vi "Initialize_Devices.vi"(6 "Queues":T3, 8 "Status/Errors in":refnum<vi>, 9 "Control Parameters [] in":T18[](array[typedef]) {"Aux Byte Value" format="%02x"; "Max Real Value" format="%#_6e"; "Min Real Value" format="%#_6e"; "dReal/dByte" format="%#_6e"; "Byte Value" format="%02x"; "Identifier" format="%02x"}, 10 "Main parameters in":T4={"Mode"={"Mode"=enum."Dialog", "Expert?"=FALSE, "Dialog?"=FALSE}, "Stop loop"={"Settings changed?"=FALSE, "Stop?"=refnum}, "Send message"={"Send mode"=enum."Get parameters", "Set parameter list"=0, "Get parameter list"=0, "Reset device"=0, "Length set settings message"=0, "Reset buttons?"=FALSE, "Reset Master?"=enum."General"}, "Write settings"={"Options"=enum."File 1"}, "Settings state"={"MAS locked?"=refnum, "SLV locked?"=refnum}, "Button refs"={"Stop program"=refnum, "Save settings"=refnum, "DAQ mode"=refnum, "Reset settings"=refnum, "Apply settings"=refnum, "Reset MAS"=refnum, "Reset SLV"=refnum, "Local DBase?"=refnum, "Last value DBase"=FALSE, "Database"=refnum, "Calibration"=refnum, "Save settings 2"=refnum}, "Update screen"={"Detector number"=0, "Hardware"=enum."None"}, "Files"={"Path config file"=path "", "Path def. ini file"=path "", "Path ini file 1"=path "", "Path ini file 2"=path "", "Path RBF file"=path ""}, "DB connection"={"connection reference"=refnum, "Connected?"=refnum, "ODBC Name"=""}, "Status_id"=refnum, "Time difference"=refnum, "Satellites"=refnum, "Alignment parameters"=refnum, "Page Statistics 2"=refnum, "Database"=refnum, "Page Statistics"=refnum} {"Update screen"."Detector number" format="%#.0f"; "Send message"."Reset device" format="%x"; "Send message"."Get parameter list" format="%x"; "Send message"."Set parameter list" format="%x"}, 11 "Timer parameters":refnum<vi>) -> (0 "Status/Errors out":refnum<vi>, 1 "Control Parameters [] out":T18[](array[typedef]) {"Aux Byte Value" format="%02x"; "Max Real Value" format="%#_6e"; "Min Real Value" format="%#_6e"; "dReal/dByte" format="%#_6e"; "Byte Value" format="%02x"; "Identifier" format="%02x"}, 2 "Main parameters out":T4={"Mode"={"Mode"=enum."Dialog", "Expert?"=FALSE, "Dialog?"=FALSE}, "Stop loop"={"Settings changed?"=FALSE, "Stop?"=refnum}, "Send message"={"Send mode"=enum."Get parameters", "Set parameter list"=0, "Get parameter list"=0, "Reset device"=0, "Length set settings message"=0, "Reset buttons?"=FALSE, "Reset Master?"=enum."General"}, "Write settings"={"Options"=enum."File 1"}, "Settings state"={"MAS locked?"=refnum, "SLV locked?"=refnum}, "Button refs"={"Stop program"=refnum, "Save settings"=refnum, "DAQ mode"=refnum, "Reset settings"=refnum, "Apply settings"=refnum, "Reset MAS"=refnum, "Reset SLV"=refnum, "Local DBase?"=refnum, "Last value DBase"=FALSE, "Database"=refnum, "Calibration"=refnum, "Save settings 2"=refnum}, "Update screen"={"Detector number"=0, "Hardware"=enum."None"}, "Files"={"Path config file"=path "", "Path def. ini file"=path "", "Path ini file 1"=path "", "Path ini file 2"=path "", "Path RBF file"=path ""}, "DB connection"={"connection reference"=refnum, "Connected?"=refnum, "ODBC Name"=""}, "Status_id"=refnum, "Time difference"=refnum, "Satellites"=refnum, "Alignment parameters"=refnum, "Page Statistics 2"=refnum, "Database"=refnum, "Page Statistics"=refnum} {"Update screen"."Detector number" format="%#.0f"; "Send message"."Reset device" format="%x"; "Send message"."Get parameter list" format="%x"; "Send message"."Set parameter list" format="%x"}, 3 "Devices":T17)   [LabVIEW 2010]
uses:
  Controls/Control_Parameters.ctl
  Controls/Master.ctl
  Controls/Devices.ctl
  Controls/Main_Parameters.ctl
  Controls/Mode.ctl
  Controls/Stop_Loop.ctl
  Controls/Send_Message.ctl
  Controls/Send_Message_Mode.ctl
  Controls/Write_Settings.ctl
  Controls/Write_Settings_Options.ctl
  Controls/Settings_State.ctl
  Controls/Button_Refs.ctl
  Controls/Update_Screen.ctl
  Controls/Files.ctl
  Controls/DB_Connection.ctl
  database/Connection.llb/Conn ObjectReference.ctl
  Controls/Queues.ctl
  Controls/One_Second.ctl
  Controls/GPS_Timestamp.ctl
  Controls/Device.ctl
  Controls/Set_Mode.ctl
  Controls/Get_Set_Connection_Options.ctl
  Controls/Get_Set_Buttons_mode.ctl
  Controls/Get_Set_Settings_State_Options.ctl
panel:
  in  "Slave":T1
  in  "Master":T1
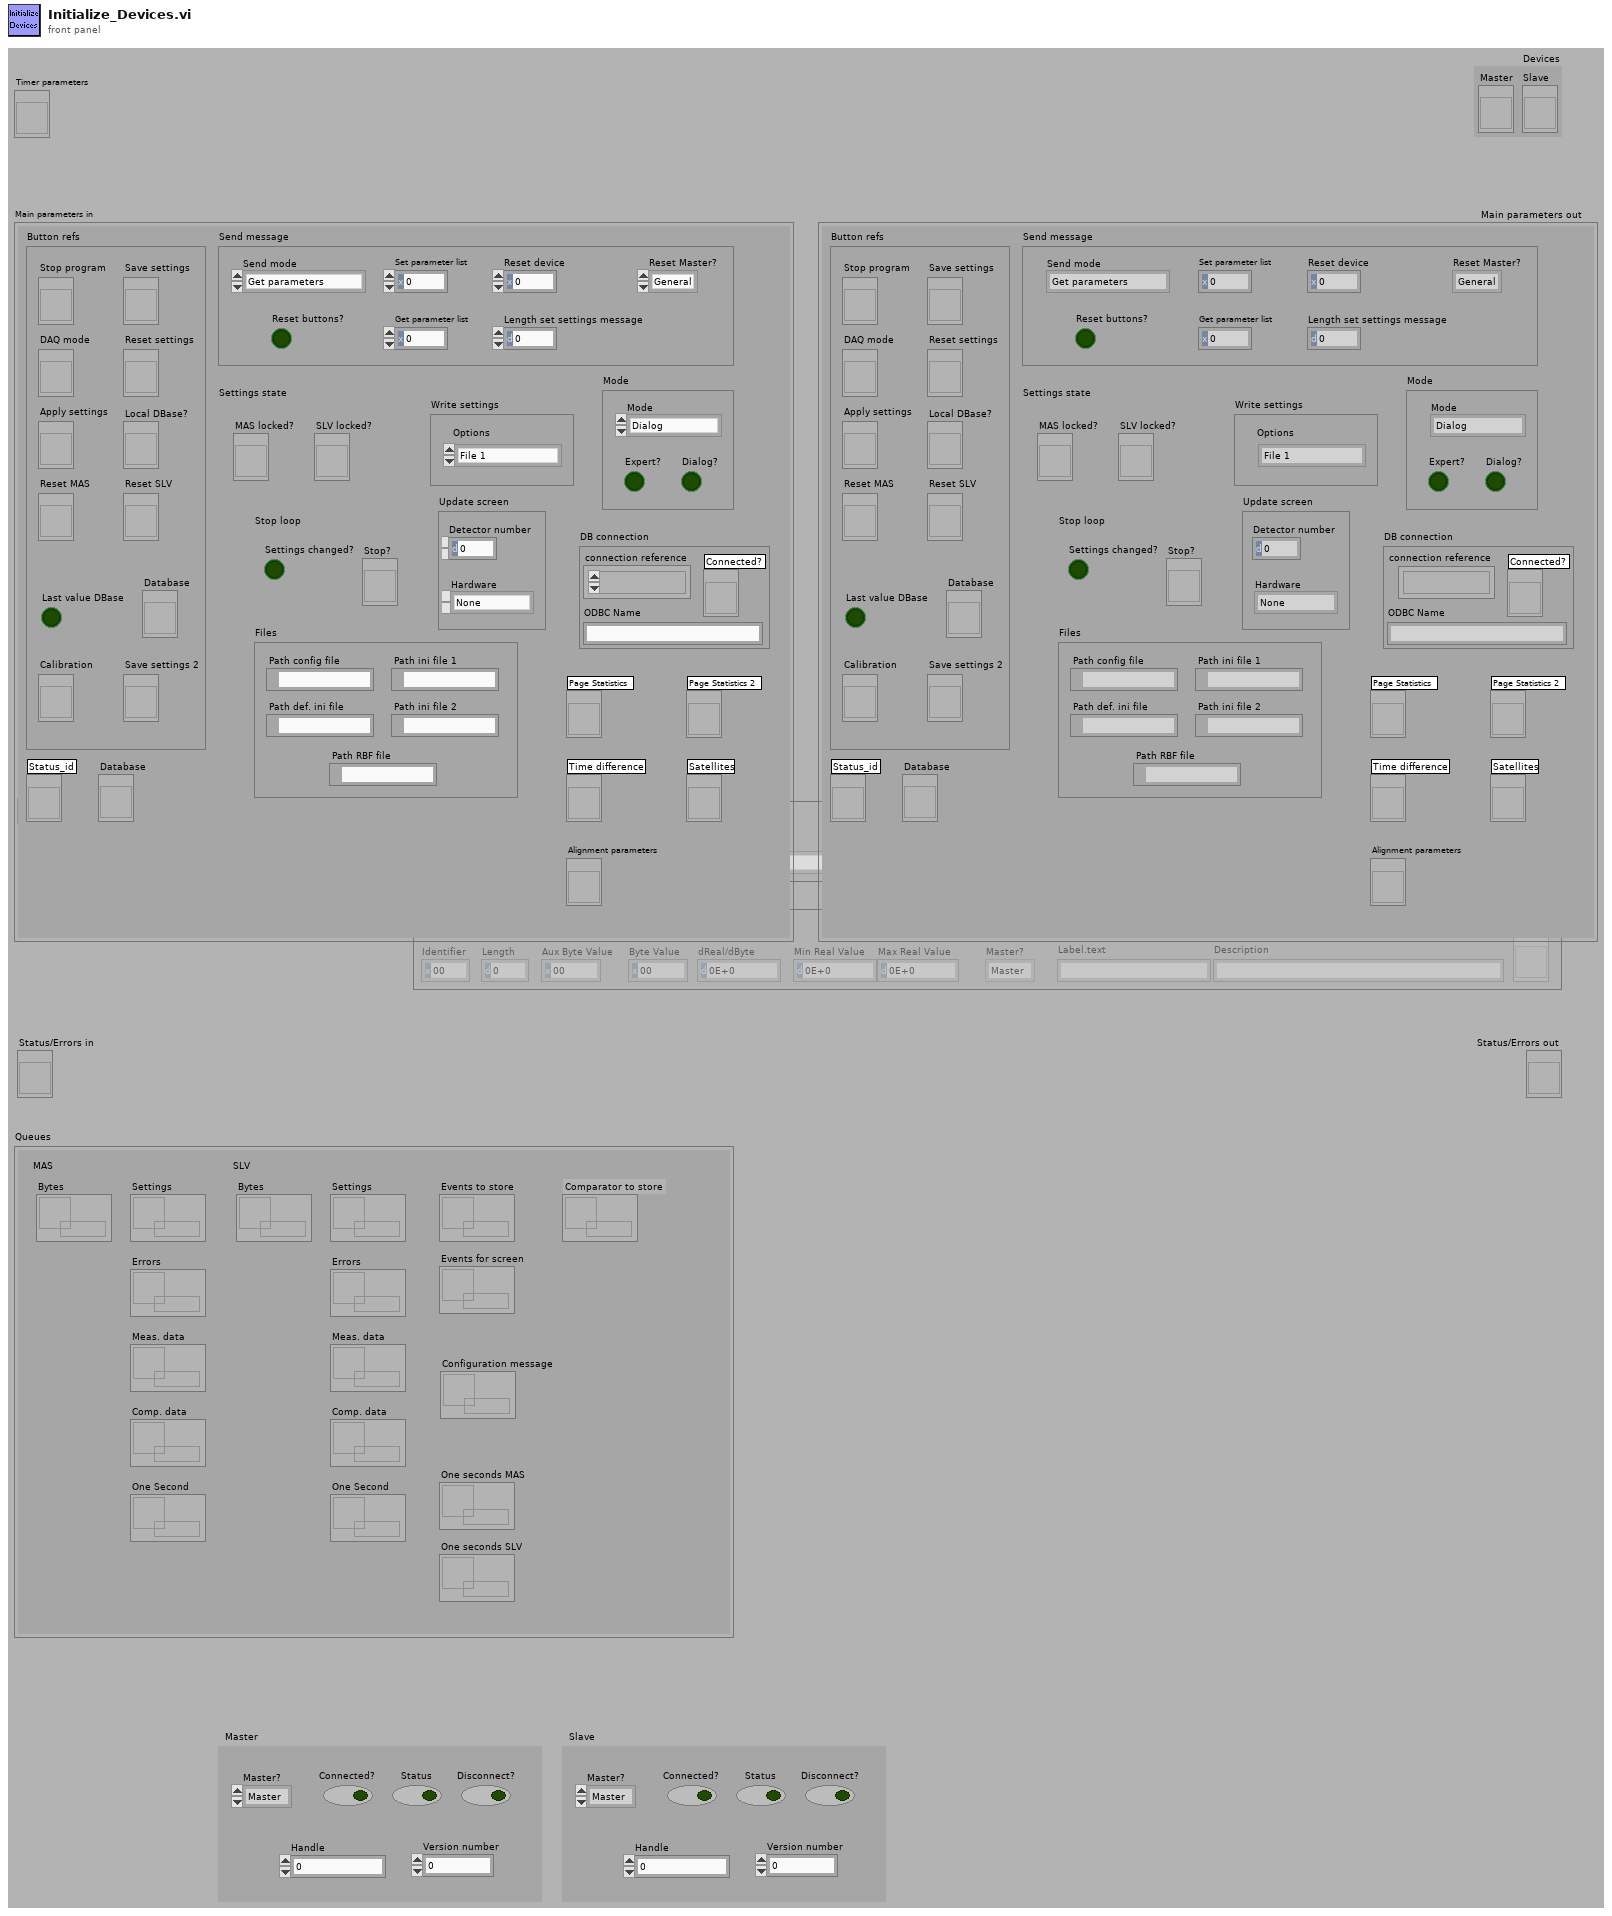
[diagram p1: front panel]
types:
  T1 = typedef "Device.ctl" = cluster{"Master?":T2, "Connected?":bool, "Status":bool, "Disconnect?":bool, "Handle":u32, "Version number":u32}
  T2 = typedef "Master.ctl" = enum16{"Master", "Slave", "General"}
  T3 = typedef "Queues.ctl" = cluster{"MAS":cluster{"Bytes":refnum<queue>, "Settings":refnum<queue>, "Errors":refnum<queue>, "Meas. data":refnum<queue>, "One Second":refnum<queue>, "Comp. data":refnum<queue>}, "SLV":cluster{"Bytes":refnum<queue>, "Settings":refnum<queue>, "Errors":refnum<queue>, "Meas. data":refnum<queue>, "One Second":refnum<queue>, "Comp. data":refnum<queue>}, "Events to store":refnum<queue>, "Events for screen":refnum<queue>, "One seconds MAS":refnum<queue>, "One seconds SLV":refnum<queue>, "Configuration message":refnum<queue>, "Comparator to store":refnum<queue>}
  T4 = typedef "Main_Parameters.ctl" = cluster{"Mode":T5, "Stop loop":T6, "Send message":T7, "Write settings":T9, "Settings state":T11, "Button refs":T12, "Update screen":T13, "Files":T14, "DB connection":T15, "Status_id":refnum<vi>, "Time difference":refnum<vi>, "Satellites":refnum<vi>, "Alignment parameters":refnum<vi>, "Page Statistics 2":refnum<vi>, "Database":refnum<vi>, "Page Statistics":refnum<vi>}
  T5 = typedef "Mode.ctl" = cluster{"Mode":enum8{"Stop", "Dialog", "Hisparc II", "Hisparc II DAQ", "Alignment"}, "Expert?":bool, "Dialog?":bool}
  T6 = typedef "Stop_Loop.ctl" = cluster{"Settings changed?":bool, "Stop?":refnum<vi>}
  T7 = typedef "Send_Message.ctl" = cluster{"Send mode":T8, "Set parameter list":u8, "Get parameter list":u8, "Reset device":u8, "Length set settings message":i32, "Reset buttons?":bool, "Reset Master?":T2}
  T8 = typedef "Send_Message_Mode.ctl" = enum16{"Get parameters", "Set parameters", "From front panel", "From parameters", "Reset device", "Alignment"}
  T9 = typedef "Write_Settings.ctl" = cluster{"Options":T10}
  T10 = typedef "Write_Settings_Options.ctl" = enum16{"File 1", "File 2", "Alignment", "Reset"}
  T11 = typedef "Settings_State.ctl" = cluster{"MAS locked?":refnum<vi>, "SLV locked?":refnum<vi>}
  T12 = typedef "Button_Refs.ctl" = cluster{"Stop program":refnum<vi>, "Save settings":refnum<vi>, "DAQ mode":refnum<vi>, "Reset settings":refnum<vi>, "Apply settings":refnum<vi>, "Reset MAS":refnum<vi>, "Reset SLV":refnum<vi>, "Local DBase?":refnum<vi>, "Last value DBase":bool, "Database":refnum<vi>, "Calibration":refnum<vi>, "Save settings 2":refnum<vi>}
  T13 = typedef "Update_Screen.ctl" = cluster{"Detector number":u16, "Hardware":enum8{"None", "HiSPARC I", "HiSPARC II", "HiSPARC III", "Unknown"}}
  T14 = typedef "Files.ctl" = cluster{"Path config file":path, "Path def. ini file":path, "Path ini file 1":path, "Path ini file 2":path, "Path RBF file":path}
  T15 = typedef "DB_Connection.ctl" = cluster{"connection reference":T16, "Connected?":refnum<vi>, "ODBC Name":string}
  T16 = typedef "Conn ObjectReference.ctl" = refnum<k1>
  T17 = typedef "Devices.ctl" = cluster{"Master":refnum<vi>, "Slave":refnum<vi>}
  T18 = typedef "Control_Parameters.ctl" = cluster{"Identifier":u8, "Length":u16, "Byte Value":u32, "dReal/dByte":dbl, "Min Real Value":dbl, "Max Real Value":dbl, "Master?":T2, "Label.text":string, "Description":string, "Refnum":refnum<vi>, "Aux Byte Value":u32}
  T19 = typedef "Get_Set_Connection_Options.ctl" = enum16{"Get", "Set connect", "Set disconnect"}
  T20 = typedef "Set_Mode.ctl" = enum16{"Create Message Only", "Front Panel", "Parameters", "Master", "Slave"}
  T21 = enum8{"None", "HiSPARC I", "HiSPARC II", "HiSPARC III", "Unknown"}
  T22 = typedef "Semaphore RefNum" = refnum<k1>
  T23 = typedef "Get_Set_Buttons_mode.ctl" = enum16{"Get", "Get DAQ", "Set", "Set settings"}
  T24 = typedef "Get_Set_Settings_State_Options.ctl" = enum16{"Get", "Lock", "Unlock"}
  T25 = typedef "Settings_Message.ctl" = T26[]
  T26 = typedef "Setting.ctl" = cluster{"Identifier":u8, "  Bytes":u8[], "# Bytes":u16}
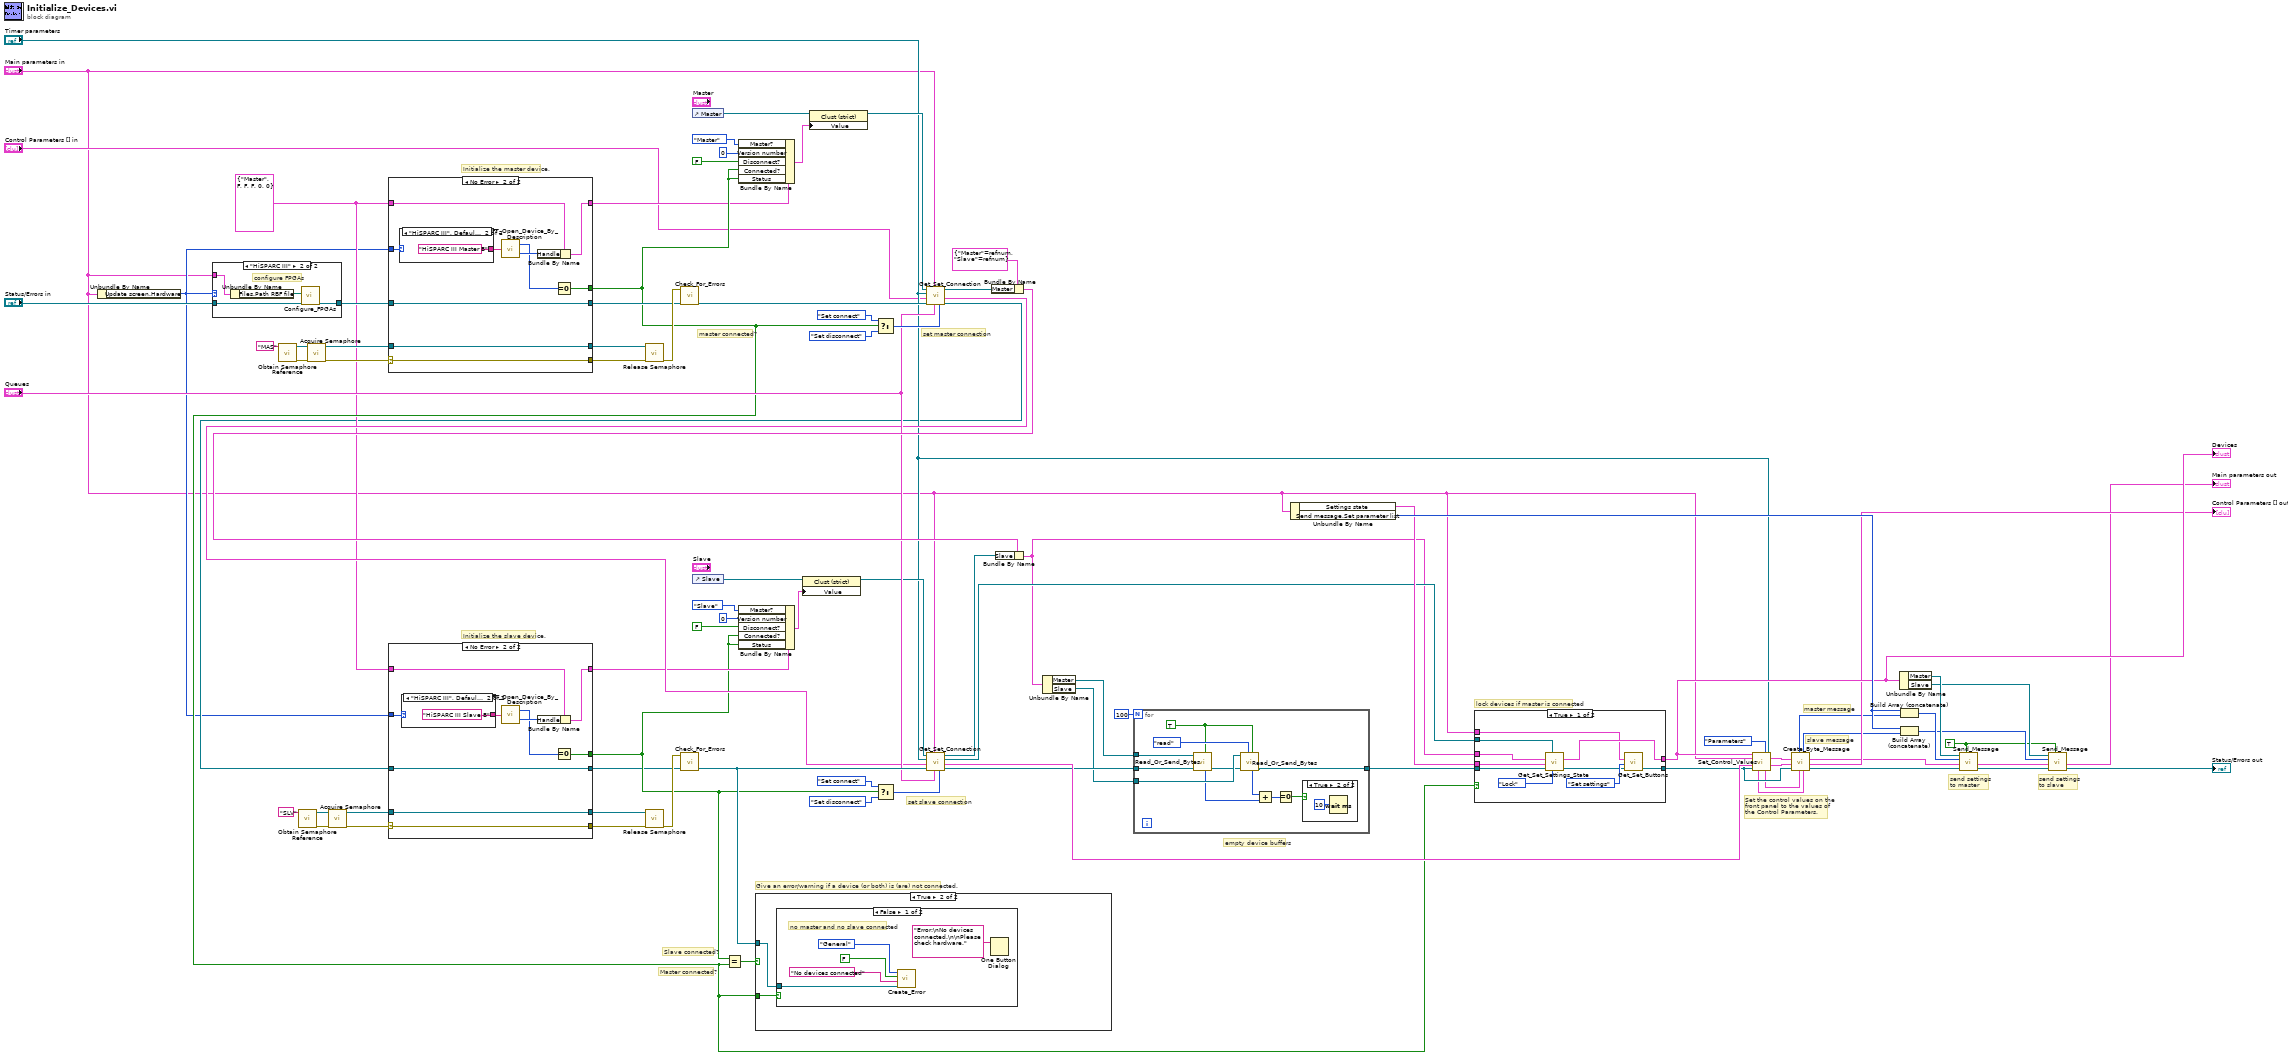
[diagram p0: block diagram]
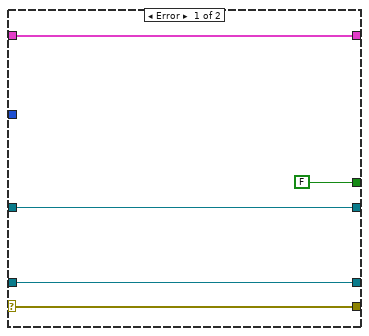
[diagram p2: hidden frame]
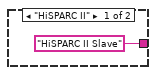
[diagram p3: hidden frame]
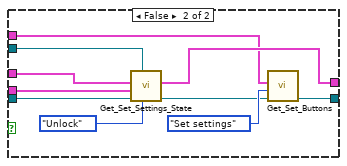
[diagram p6: hidden frame]
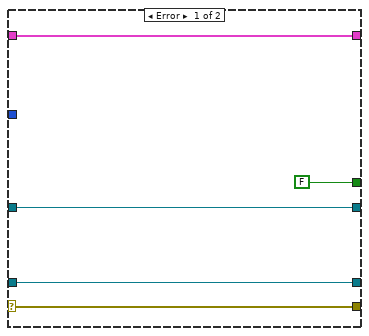
[diagram p7: hidden frame]
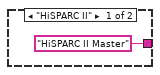
[diagram p8: hidden frame]
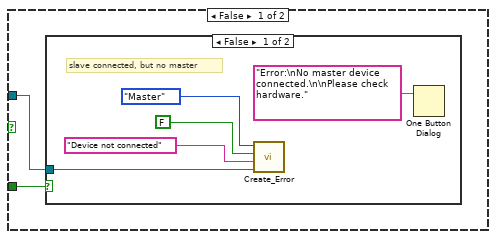
[diagram p9: hidden frame]
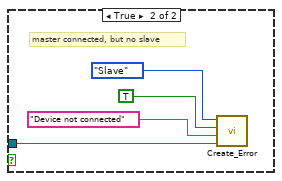
[diagram p10: hidden frame]
diagram:
  w13 = T1 {"Master?"=enum."Master", "Connected?"=FALSE, "Status"=FALSE, "Disconnect?"=FALSE, "Handle"=0, "Version number"=0} ("Master")
  w57 = TRUE ("Ask Parameter Message? (false)")
  # "empty device buffers"
  # "lock devices if master is connected"
  # "Initialize the master device."
  # "Initialize the slave device."
  # "send settings\nto slave"
  # "send settings\nto master"
  # "slave message"
  # "master message"
  # "Set the control values on the\nfront panel to the values of\nthe Control Parameters."
  # "set slave connection"
  # "master connected?"
  # "set master connection"
  # "Give an error/warning if a device (or both) is (are) not connected."
  # "Master connected?"
  # "Slave connected?"
  n1 = Unbundle By Name("Main parameters in") -> ("Update screen.Hardware"=w2:T21)
  n2 = case shown="\"HiSPARC III\"" w2 {
    tunnel: "Status/Errors in" -> [w89 w93]
    tunnel: [w89 w92] -> w17
    tunnel: "Main parameters in" -> [_ w91]
    frame Default {
    }
    frame "HiSPARC III" {
      # "configure FPGAs"
      n3 = Unbundle By Name(w91) -> ("Files.Path RBF file"=w90:path)
      n4 = call "Configure_FPGAs.vi"("Status/Errors in"=w93, "RBF file path in"=w90) -> ("Status/Errors out"=w92:refnum<vi>)  [unwired: 9 out]
    }
  }
  n5 = call <vilib>:"Obtain Semaphore Reference.vi"("name (unnamed)"="MAS") -> ("error out"=w71:errorcluster, "semaphore"=w73:T22)  [unwired: 2 in, 3 out]
  n6 = call <vilib>:"Obtain Semaphore Reference.vi"("name (unnamed)"="SLV") -> ("error out"=w68:errorcluster, "semaphore"=w70:T22)  [unwired: 2 in, 3 out]
  n7 = call <vilib>:"Acquire Semaphore.vi"("error in (no error)"=w71, "semaphore"=w73) -> ("error out"=w30:errorcluster, "semaphore out"=w46:T22)  [unwired: 1 in, 3 out]
  n8 = call <vilib>:"Acquire Semaphore.vi"("error in (no error)"=w68, "semaphore"=w70) -> ("error out"=w12:errorcluster, "semaphore out"=w10:T22)  [unwired: 1 in, 3 out]
  n9 = case shown="No Error" w30 {
    selector: w30 -> [w94 w101]
    tunnel: w13 -> [w97 w107]
    tunnel: [w97 w106] -> w41
    tunnel: [FALSE w103] -> w42
    tunnel: w17 -> [w96 w105]
    tunnel: [w96 w105] -> w49
    tunnel: w46 -> [w95 w108]
    tunnel: [w95 w108] -> w48
    tunnel: [w94 w101] -> w47
    tunnel: w2 -> [_ w99]
    frame Error {
    }
    frame No Error {
      n10 = case shown="\"HiSPARC III\", Default" w99 {
        tunnel: ["HiSPARC II Master" ("Device Description") "HiSPARC III Master B" ("Device Description")] -> w100
        frame "HiSPARC II" {
        }
        frame "HiSPARC III", Default {
        }
      }
      n11 = call "FT_Open_Device_By_Description.vi"("Device Description"=w100) -> ("FT_Status"=w102:u32, "Handle"=w104:u32)
      n12 = Bundle By Name(cluster=w107, "Handle"=w104) -> (w106:T1)
      n13 = Equal To 0?(x=w102) -> (x = 0?=w103:bool)
    }
  }
  n14 = call <vilib>:"Release Semaphore.vi"("error in (no error)"=w47, "semaphore"=w48) -> ("error out"=w66:errorcluster)  [unwired: 5 out]
  n15 = call "Check_For_Errors.vi"("Status/Errors in"=w49, "error in"=w66) -> ("Status/Errors out"=w67:refnum<vi>)  [unwired: 9 out]
  n16 = control-ref of="Master"() -> (w28:refnum<vi>)
  n17 = control-ref of="Slave"() -> (w29:refnum<vi>)
  n18 = Bundle By Name(cluster=w41, "Master?"=Master."Master", "Version number"=u32 0 ("Master.device id"), "Disconnect?"=FALSE, "Connected?"=w42, "Status"=w42) -> (w62:T1)
  n19 = property class="Clust (strict)"(reference=w28, "Value"=w62) -> (reference out=w32:refnum<vi>)  [unwired: 1 in, 1 out]
  n20 = Select(t=Get_Set_Connection_Options."Set connect" ("Get/Set"), s=w42, f=Get_Set_Connection_Options."Set disconnect") -> (s? t:f=w51:T19)
  n21 = call "Get_Set_Connection.vi"("Get/Set"=w51, "Queues"="Queues", "Main parameters in"="Main parameters in", "Status/Errors in"=w67, "Control Parameters [] in"="Control Parameters [] in", "Timer parameters in"="Timer parameters", "Device in"=w32) -> ("Status/Errors out"=w11:refnum<vi>, "Control Parameters [] out"=w31:T18[], "Device out"=w76:refnum<vi>)  [unwired: 2 out]
  n22 = case shown="No Error" w12 {
    selector: w12 -> [w111 w118]
    tunnel: w13 -> [w114 w124]
    tunnel: [w114 w123] -> w9
    tunnel: [FALSE w120] -> w8
    tunnel: w11 -> [w113 w122]
    tunnel: [w113 w122] -> w7
    tunnel: w10 -> [w112 w125]
    tunnel: [w112 w125] -> w6
    tunnel: [w111 w118] -> w5
    tunnel: w2 -> [_ w116]
    frame Error {
    }
    frame No Error {
      n23 = case shown="\"HiSPARC III\", Default" w116 {
        tunnel: ["HiSPARC II Slave" ("Device Description") "HiSPARC III Slave B" ("Device Description")] -> w117
        frame "HiSPARC II" {
        }
        frame "HiSPARC III", Default {
        }
      }
      n24 = call "FT_Open_Device_By_Description.vi"("Device Description"=w117) -> ("FT_Status"=w119:u32, "Handle"=w121:u32)
      n25 = Bundle By Name(cluster=w124, "Handle"=w121) -> (w123:T1)
      n26 = Equal To 0?(x=w119) -> (x = 0?=w120:bool)
    }
  }
  n27 = call <vilib>:"Release Semaphore.vi"("error in (no error)"=w5, "semaphore"=w6) -> ("error out"=w64:errorcluster)  [unwired: 5 out]
  n28 = call "Check_For_Errors.vi"("Status/Errors in"=w7, "error in"=w64) -> ("Status/Errors out"=w65:refnum<vi>)  [unwired: 9 out]
  n29 = Equal?(x=w8, y=w42) -> (x = y?=w86:bool)
  n30 = Bundle By Name(cluster=w9, "Master?"=Master."Slave", "Version number"=u32 0 ("Master.device id"), "Disconnect?"=FALSE, "Connected?"=w8, "Status"=w8) -> (w58:T1)
  n31 = case shown="True" w86 {
    tunnel: w65 -> [w128 w139]
    tunnel: w42 -> [w129 w140]
    frame False {
      n32 = case shown="False" w129 {
        tunnel: w128 -> [w131 w135]
        frame False {
          # "slave connected, but no master"
          n33 = call "Create_Error.vi"("Status/Errors in"=w131, "HiSPARC error"="Device not connected", "Warning? (false)"=FALSE, "Master?"=Master."Master") -> ()  [unwired: 2 in, 6 out]
          n34 = One Button Dialog(message="Error:\nNo master device connected.\n\nPlease check hardware.") -> ()  [unwired: 2 out]
        }
        frame True {
          # "master connected, but no slave"
          n35 = call "Create_Error.vi"("Status/Errors in"=w135, "HiSPARC error"="Device not connected", "Warning? (false)"=TRUE, "Master?"=Master."Slave") -> ()  [unwired: 2 in, 6 out]
        }
      }
    }
    frame True {
      n36 = case shown="False" w140 {
        tunnel: w139 -> [w142 _]
        frame False {
          # "no master and no slave connected"
          n37 = call "Create_Error.vi"("Status/Errors in"=w142, "HiSPARC error"="No devices connected", "Warning? (false)"=FALSE, "Master?"=Master."General") -> ()  [unwired: 2 in, 6 out]
          n38 = One Button Dialog(message="Error:\nNo devices connected.\n\nPlease check hardware.") -> ()  [unwired: 2 out]
        }
        frame True {
          # "both master and slave connected"
        }
      }
    }
  }
  n39 = property class="Clust (strict)"(reference=w29, "Value"=w58) -> (reference out=w33:refnum<vi>)  [unwired: 1 in, 1 out]
  n40 = Select(t=Get_Set_Connection_Options."Set connect" ("Get/Set"), s=w8, f=Get_Set_Connection_Options."Set disconnect") -> (s? t:f=w54:T19)
  n41 = call "Get_Set_Connection.vi"("Get/Set"=w54, "Queues"="Queues", "Main parameters in"="Main parameters in", "Status/Errors in"=w65, "Control Parameters [] in"=w31, "Timer parameters in"="Timer parameters", "Device in"=w33) -> ("Status/Errors out"=w38:refnum<vi>, "Control Parameters [] out"=w45:T18[], "Timer parameters out"=w39:refnum<vi>, "Device out"=w75:refnum<vi>)  [unwired: 1 out]
  n42 = Bundle By Name(cluster=T17 {"Master"=refnum, "Slave"=refnum} ("Devices"), "Master"=w76) -> (w84:T17)
  n43 = Bundle By Name(cluster=w84, "Slave"=w75) -> (w36:T17)
  n44 = Unbundle By Name(w36) -> ("Master"=w35:refnum<vi>, "Slave"=w34:refnum<vi>)
  n45 = for {
    N: 100 -> [_]
    tunnel: w35 -> [w150]
    tunnel: w34 -> [w154]
    tunnel: w38 -> [w147]
    tunnel: [w153] -> w37
    w149 = TRUE ("Aquire semaphore? (t)")
    n46 = call "Read_Or_Send_Bytes.vi"("Aquire semaphore? (t)"=w149, "Status/Errors in"=w147, "Device in"=w150) -> ("Status/Errors out"=w146:refnum<vi>, "Bytes at Port"=w148:u32)  [unwired: 2 in, 5 out]
    n47 = call "Read_Or_Send_Bytes.vi"("Aquire semaphore? (t)"=w149, "Read or write?"=enum8{"read", "write"}."read", "Status/Errors in"=w146, "Device in"=w154) -> ("Status/Errors out"=w153:refnum<vi>, "Bytes at Port"=w152:u32)  [unwired: 1 in, 5 out]
    n48 = Add(x=w152, y=w148) -> (x+y=w156:u32)
    n49 = Equal To 0?(x=w156) -> (x = 0?=w155:bool)
    n50 = case shown="True" w155 {
      frame False {
      }
      frame True {
        n51 = Wait (ms)(milliseconds to wait=u32 10) -> ()  [unwired: 1 out]
      }
    }
  }
  n52 = Unbundle By Name("Main parameters in") -> ("Settings state"=w44:T11, "Send message.Set parameter list"=w79:u8)
  n53 = case shown="True" w42 {
    tunnel: w44 -> [w167 w177]
    tunnel: w37 -> [w166 w176]
    tunnel: [w161 w171] -> w25
    tunnel: w36 -> [w165 w175]
    tunnel: w39 -> [w164 w174]
    tunnel: [w159 w169] -> w43
    tunnel: "Main parameters in" -> [w158 w168]
    frame True {
      n54 = call "Get_Set_Settings_State.vi"("Get/Set"=Get_Set_Settings_State_Options."Lock", "Timer parameters"=w164, "Status/Errors in"=w166, "Settings state"=w167, "Devices in"=w165) -> ("Status/Errors out"=w160:refnum<vi>, "Devices out"=w159:T17)  [unwired: 5 out]
      n55 = call "Get_Set_Buttons.vi"("Status/Errors in"=w160, "Set?"=Get_Set_Buttons_mode."Set settings", "Main parameters"=w158) -> ("Status/Errors out"=w161:refnum<vi>)  [unwired: 1 in, 7 out]
    }
    frame False {
      n56 = call "Get_Set_Settings_State.vi"("Get/Set"=Get_Set_Settings_State_Options."Unlock", "Timer parameters"=w174, "Status/Errors in"=w176, "Settings state"=w177, "Devices in"=w175) -> ("Status/Errors out"=w170:refnum<vi>, "Devices out"=w169:T17)  [unwired: 5 out]
      n57 = call "Get_Set_Buttons.vi"("Status/Errors in"=w170, "Set?"=Get_Set_Buttons_mode."Set settings", "Main parameters"=w168) -> ("Status/Errors out"=w171:refnum<vi>)  [unwired: 1 in, 7 out]
    }
  }
  "Devices" <- w43
  n58 = call "Set_Control_Values.vi"("Devices in"=w43, "Set Mode"=Set_Mode."Parameters", "Timer parameters in"="Timer parameters", "Main Parameters in"="Main parameters in", "Control Parameters [] in"=w45, "Status/Errors in"=w25) -> ("Main parameters out"=w27:T4, "Control Parameters [] out"=w26:T18[], "Slave Settings Message"=w21:T25, "Master Settings Message"=w22:T25)  [unwired: 1 in, 5 out]
  n59 = call "Create_Byte_Message.vi"("Slave Settings Message in"=w21, "Master Settings Message in"=w22, "Status/Errors in"=w25, "Control Parameters [] in"=w26, "Main Parameters in"=w27) -> ("Status/Errors out"=w24:refnum<vi>, "Control Parameters [] out"=→"Control Parameters [] out":T18[], "Main parameters out"=w15:T4, "Slave Byte Message out"=w19:u8[], "Master Byte Message out"=w20:u8[])  [unwired: 2 out]
  n60 = Unbundle By Name(w43) -> ("Master"=w81:refnum<vi>, "Slave"=w80:refnum<vi>)
  n61 = Build Array (concatenate)(w79, w20) -> (w78:u8[])
  n62 = Build Array (concatenate)(w79, w19) -> (w77:u8[])
  n63 = call "Send_Message.vi"("Ask Parameter Message? (false)"=w57, "Status/Errors in"=w24, "Main parameters in"=w15, "Byte Message"=w78, "Device in"=w81) -> ("Status/Errors out"=w83:refnum<vi>, "Main parameters out"=w82:T4)  [unwired: 5 out]
  n64 = call "Send_Message.vi"("Ask Parameter Message? (false)"=w57, "Status/Errors in"=w83, "Main parameters in"=w82, "Byte Message"=w77, "Device in"=w80) -> ("Status/Errors out"=→"Status/Errors out":refnum<vi>, "Main parameters out"=→"Main parameters out":T4)  [unwired: 5 out]
